vi "winForms keyDownResponse.vi"(4 "searchString":refnum<vi>, 6 "editorType":T1=enum."SigProc", 7 "Ctrl":bool, 8 "error in (no error)":errorcluster, 9 "Char":i16, 10 "VKey":T2, 11 "scintillaRefNum":refnum<k24>) -> (0 "error out":errorcluster, 1 "Discard?":bool)   [LabVIEW 2018]
uses:
  <vilib>/event_ctls.llb/eventvkey.ctl
  C:/ATI_MS_InstrumentControl/dll/ScintillaNET.dll
  dll/ScintillaNET.dll
  winForms editorType.ctl
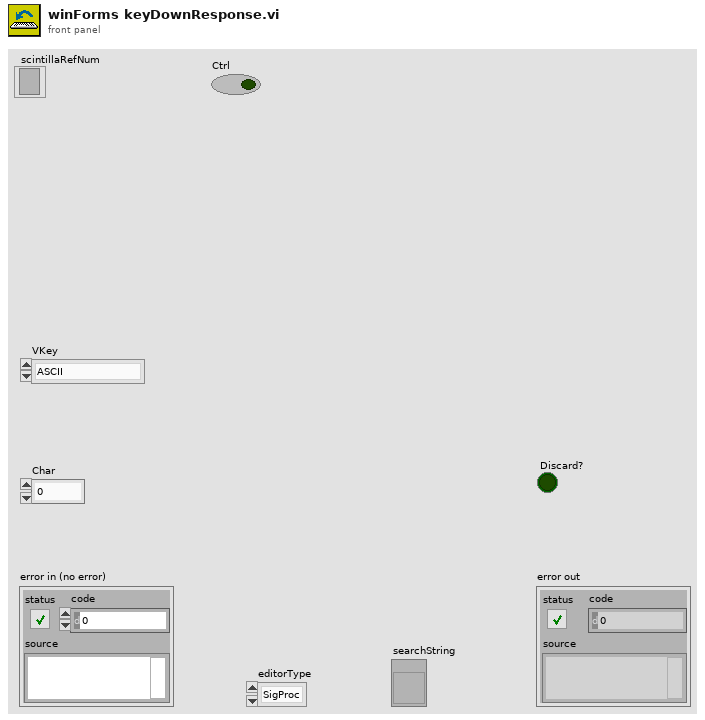
[diagram p1: front panel]
types:
  T1 = typedef "winForms editorType.ctl" = enum16{"Recipe", "SigProc", "Editor"}
  T2 = typedef "eventvkey.ctl" = enum16{"ASCII", "Enter", "Return", "Shift", "Ctrl", "Alt", "Cmd", "Opt", "Caps", "NumLock", "Clear", "Break", "Up", "Down", "Left", "Right", "Insert", "Delete", "Home", "End", "PageUp", "PageDown", "Escape", "Help", "Pause", "ScrollLock", "F1", "F2", "F3", "F4", "F5", "F6", "F7", "F8", "F9", "F10", "F11", "F12", "F13", "F14", "F15", "F16", "F17", "F18", "F19", "F20", "F21", "F22", "F23", "F24", "Play", "VolumeUp", "VolumeDown", "Mute", "Two Byte Char"}
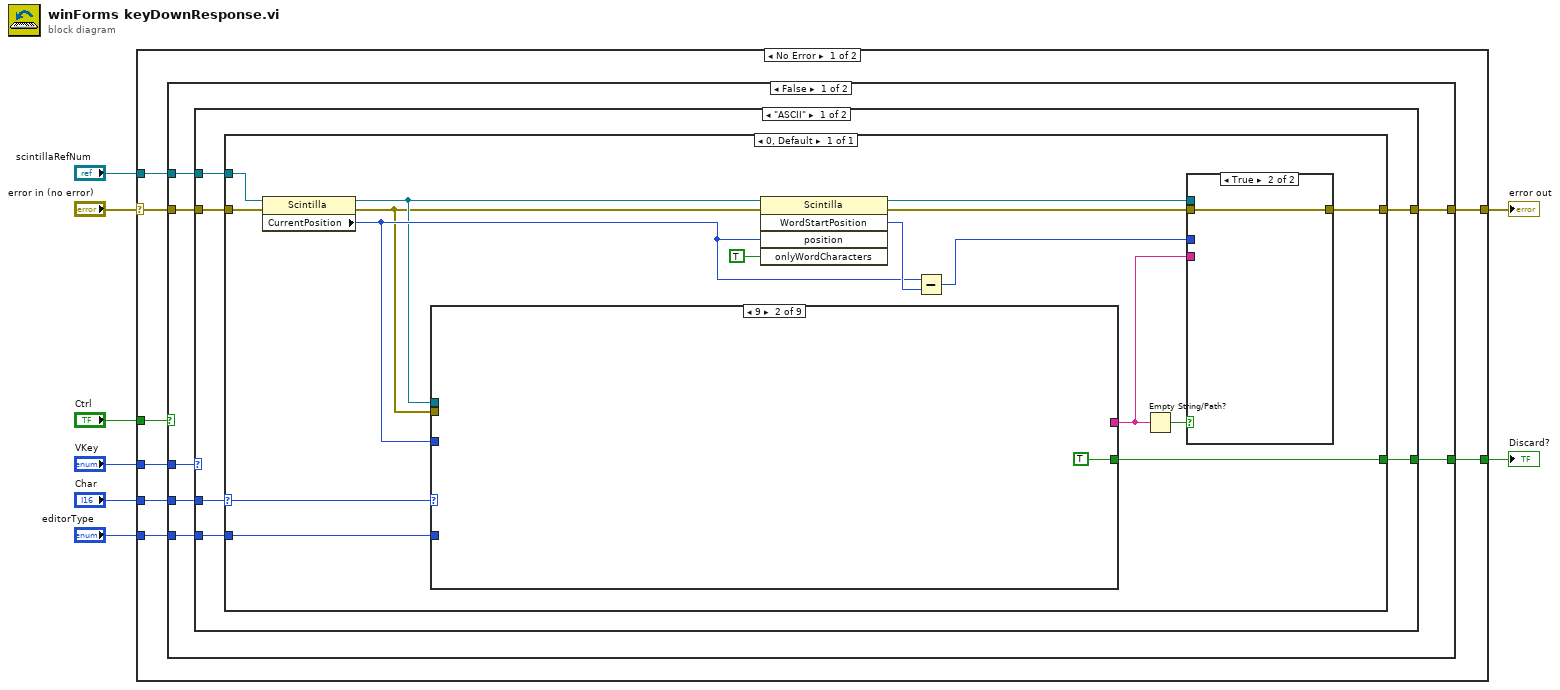
[diagram p0: block diagram]
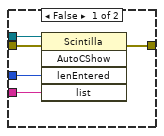
[diagram p2: hidden frame]
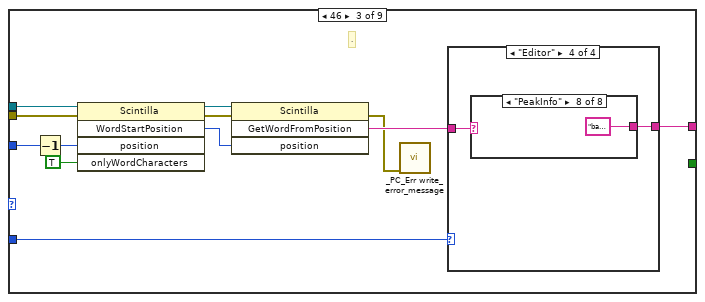
[diagram p4: hidden frame]
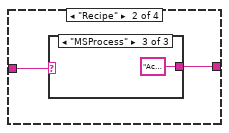
[diagram p6: hidden frame]
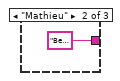
[diagram p8: hidden frame]
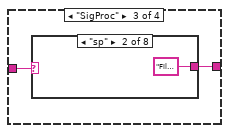
[diagram p9: hidden frame]
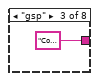
[diagram p11: hidden frame]
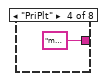
[diagram p12: hidden frame]
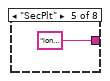
[diagram p13: hidden frame]
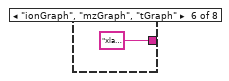
[diagram p14: hidden frame]
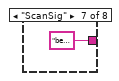
[diagram p15: hidden frame]
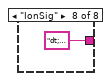
[diagram p16: hidden frame]
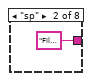
[diagram p18: hidden frame]
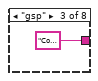
[diagram p19: hidden frame]
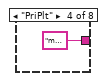
[diagram p20: hidden frame]
diagram:
  n1 = case shown="No Error" "error in (no error)" {
    selector: "error in (no error)" -> [w13 w123]
    tunnel: "VKey" -> [w16 _]
    tunnel: "Char" -> [w15 _]
    tunnel: "scintillaRefNum" -> [w14 _]
    tunnel: [w12 w123] -> w4
    tunnel: [w11 _] -> w3
    tunnel: "editorType" -> [w10 _]
    tunnel: "Ctrl" -> [w9 _]
    frame No Error {
      n2 = case shown="False" w9 {
        tunnel: w16 -> [w23 _]
        tunnel: w15 -> [w22 w110]
        tunnel: w14 -> [w21 w109]
        tunnel: w13 -> [w20 w108]
        tunnel: [w19 w111] -> w12
        tunnel: [w18 TRUE] -> w11
        tunnel: w10 -> [w17 _]
        frame False {
          n3 = case shown="\"ASCII\"" w23 {
            tunnel: w21 -> [w29 _]
            tunnel: w20 -> [w28 w107]
            tunnel: w22 -> [w27 _]
            tunnel: [w26 TRUE] -> w18
            tunnel: [w25 w107] -> w19
            tunnel: w17 -> [w24 _]
            frame "ASCII" {
              n4 = case shown="0, Default" w27 {
                selector: w27 -> [w41]
                tunnel: w29 -> [w37]
                tunnel: w28 -> [w35]
                tunnel: [w30] -> w26
                tunnel: [w36] -> w25
                tunnel: w24 -> [w31]
                frame 0, Default {
                  n5 = property class="Scintilla"(reference=w37, error in=w35) -> (reference out=w33:refnum<k24>, error out=w32:errorcluster, "CurrentPosition"=w34:i32)
                  n6 = case shown="9" w41 {
                    tunnel: [_ _ w64 w87 w90 w93 w96 w100 w103] -> w38
                    tunnel: w34 -> [_ _ w61 _ _ _ _ _ _]
                    tunnel: w33 -> [_ _ w60 _ _ _ _ _ _]
                    tunnel: w32 -> [_ _ w59 _ _ _ _ _ _]
                    tunnel: w31 -> [_ _ w53 w88 w91 w94 w97 w101 w104]
                    tunnel: [_ TRUE _ _ _ _ _ _ _] -> w30
                    frame 0, Default {
                    }
                    frame 9 {
                    }
                    frame 46 {
                      # "."
                      n7 = Decrement(x=w61) -> (x-1=w62:i32)
                      n8 = invoke class="Scintilla" method="WordStartPosition"(reference=w60, error in=w59, "position"=w62, "onlyWordCharacters"=TRUE) -> (reference out=w58:refnum<k24>, error out=w57:errorcluster, "WordStartPosition"=w56:i32)  [unwired: 1 in, 2 out]
                      n9 = invoke class="Scintilla" method="GetWordFromPosition"(reference=w58, error in=w57, "position"=w56) -> (error out=w54:errorcluster, "GetWordFromPosition"=w55:string)  [unwired: 1 in, 2 out]
                      n10 = call "_PC_Err write_error_message.vi"("error in"=w54) -> ()  [unwired: 10 in, 1 out]
                      n11 = case shown="\"Editor\"" w53 {
                        tunnel: [_ w66 w69 w78] -> w64
                        tunnel: w55 -> [_ w65 w70 w79]
                        frame Default {
                        }
                        frame "Recipe" {
                          n12 = case shown="\"MSProcess\"" w65 {
                            tunnel: [_ "Betaofq(q);GetAmp( mz, freq, beta );GetBeta( mz, amp, freq );GetFreq( mz, amp, beta );GetMZ( amp, freq, beta );qofBeta( beta )" "AcqSig( time );AuxScan( auxWfmType, auxStart, iauxCyc, auxCyc, beta, betaScale, auxAmp, auxPulse1, auxPulse2, auxPulseAmp, time );CLFreqScan( targetfreq, time );FGen( amp, freq );Header( ionTrapR0, ionTrapZ0, priRFMaxAmp );IonGate( trialTime, TPH, enableAGC );LaserTrig( trigFreq, phaseDeg, shots );LinearAmpScan( auxWfmType, iauxCyc, beta, betaScale, auxAmp, auxPulse1, auxPulse2, auxPulseAmp, time, amp, continuous );PhaseScan( auxWfmType, auxStart, iauxCyc, auxCyc, beta, betaScale, auxAmp, auxPulse1, auxPulse2, auxPulseAmp, time, freq, stepWidth );PhaseScanII( auxWfmType, auxStart, iauxCyc, auxCyc, beta, betaScale, auxAmp, auxPulse1, auxPulse2, auxPulseAmp, dm, freq, stepWidth );ResetRFPhase( iniPhase );RFStart( freq, amp, wfmType );RFStop();SetDAQ( channel, sampRate );UpdAO( func, val );UpdAuxArbPulses( cycleIni, cycleEnd, pulseInt );UpdConj( iniPhase, conjLen, phaseDiff, fixedLen );UpdDO( func, val );UpdIGVolts( onVolt, offVolt );UpdRFChBias( ch1, ch2, ch3 );UpdRFChFunc( ch1, ch2, ch3 );UpdRFChScale( ch1, ch2, ch3 );Wait( timeout, DI, edge )"] -> w66
                            frame Default {
                            }
                            frame "Mathieu" {
                            }
                            frame "MSProcess" {
                            }
                          }
                        }
                        frame "SigProc" {
                          n13 = case shown="\"sp\"" w70 {
                            tunnel: [_ "Filtering( dt, ydata, ktype, kwidth );MakeKernel( dt, ktype, kwidth );NumRectifier( dt, ydata );NumRectifier_SG( dt, ydata, winwidth );PltAbs( pltData );PltFFT( pltData );PltFiltering( pltData, ktype, kwidth );PltNeg( pltData );PltNumRectifier( pltData );PltNumRectifier_SG( pltData, winwidth )" "Conv1D( kernel, ydata );PltConv1D( kernel , pltData )" "mzGraph;ScanSig;tGraph" "ionGraph;IonSig" "xlabel;ylabel" "beta;dt;xdata;ydata" "dt;ydata"] -> w69
                            frame Default {
                            }
                            frame "sp" {
                            }
                            frame "gsp" {
                            }
                            frame "PriPlt" {
                            }
                            frame "SecPlt" {
                            }
                            frame "ionGraph", "mzGraph", "tGraph" {
                            }
                            frame "ScanSig" {
                            }
                            frame "IonSig" {
                            }
                          }
                        }
                        frame "Editor" {
                          n14 = case shown="\"PeakInfo\"" w79 {
                            tunnel: [_ "Filtering( dt, ydata, ktype, kwidth );MakeKernel( dt, ktype, kwidth );NumRectifier( dt, ydata );NumRectifier_SG( dt, ydata, winwidth );PltAbs( pltData );PltFFT( pltData );PltFiltering( pltData, ktype, kwidth );PltNeg( pltData );PltNumRectifier( pltData );PltNumRectifier_SG( pltData, winwidth )" "Conv1D( kernel, ydata );PltConv1D( kernel , pltData )" "mzGraph;ScanSig;tGraph" "PeakInfo" "xlabel;ylabel" "beta;dt;xdata;ydata" "baseline;halfHeight;xCdata;xLdata;xRdata"] -> w78
                            frame Default {
                            }
                            frame "sp" {
                            }
                            frame "gsp" {
                            }
                            frame "PriPlt" {
                            }
                            frame "PeakPlt" {
                            }
                            frame "ionGraph", "mzGraph", "tGraph" {
                            }
                            frame "ScanSig" {
                            }
                            frame "PeakInfo" {
                            }
                          }
                        }
                      }
                    }
                    frame 71, 103 {
                      # "g,G"
                      n15 = case shown="\"SigProc\"" w88 {
                        tunnel: ["gsp" ("list") _] -> w87
                        frame "SigProc" {
                        }
                        frame Default {
                        }
                      }
                    }
                    frame 73, 105 {
                      # "I,i"
                      n16 = case shown="\"Recipe\"" w91 {
                        tunnel: ["instr" ("list") _] -> w90
                        frame "Recipe" {
                        }
                        frame Default {
                        }
                      }
                    }
                    frame 77, 109 {
                      # "m,M"
                      n17 = case shown="\"Recipe\"" w94 {
                        tunnel: ["Mathieu;MSProcess" ("list") _] -> w93
                        frame "Recipe" {
                        }
                        frame Default {
                        }
                      }
                    }
                    frame 80, 112 {
                      # "p,P"
                      n18 = case shown="\"SigProc\"" w97 {
                        tunnel: ["PriPlt" ("list") "PeakPlt;PriPlt" ("list") _] -> w96
                        frame "SigProc" {
                        }
                        frame "Editor" {
                        }
                        frame Default {
                        }
                      }
                    }
                    frame 83, 115 {
                      # "s,S"
                      n19 = case shown="\"SigProc\"" w101 {
                        tunnel: ["SecPlt;sp" ("list") _] -> w100
                        frame "SigProc" {
                        }
                        frame Default {
                        }
                      }
                    }
                    frame 85, 117 {
                      # "U,u"
                      n20 = case shown="\"Recipe\"" w104 {
                        tunnel: ["user" ("list") _] -> w103
                        frame "Recipe" {
                        }
                        frame Default {
                        }
                      }
                    }
                  }
                  n21 = invoke class="Scintilla" method="WordStartPosition"(reference=w33, error in=w32, "position"=w34, "onlyWordCharacters"=TRUE) -> (reference out=w45:refnum<k24>, error out=w44:errorcluster, "WordStartPosition"=w40:i32)  [unwired: 1 in, 2 out]
                  n22 = Subtract(x=w34, y=w40) -> (x-y=w42:i32)
                  n23 = Empty String/Path?(string/path=w38) -> (empty?=w39:bool)
                  n24 = case shown="True" w39 {
                    tunnel: w45 -> [w50 _]
                    tunnel: w44 -> [w49 w51]
                    tunnel: w42 -> [w48 _]
                    tunnel: w38 -> [w47 _]
                    tunnel: [w46 w51] -> w36
                    frame False {
                      n25 = invoke class="Scintilla" method="AutoCShow"(reference=w50, error in=w49, "lenEntered"=w48, "list"=w47) -> (error out=w46:errorcluster)  [unwired: 1 in, 4 out]
                    }
                    frame True {
                    }
                  }
                }
              }
            }
            frame "Enter", Default {
            }
          }
        }
        frame True {
          n26 = case shown="102" w110 {
            tunnel: w109 -> [w114 w120]
            tunnel: w108 -> [w113 w119]
            tunnel: [w115 w122] -> w111
            frame 0, Default {
              n27 = invoke class="Scintilla" method="BeginUndoAction"(reference=w114, error in=w113) -> (reference out=w116:refnum<k24>, error out=w117:errorcluster)  [unwired: 1 in, 1 out]
              n28 = invoke class="Scintilla" method="EndUndoAction"(reference=w116, error in=w117) -> (error out=w115:errorcluster)  [unwired: 1 in, 2 out]
            }
            frame 102 {
              n29 = invoke class="Scintilla" method="Undo"(reference=w120, error in=w119) -> (error out=w118:errorcluster)  [unwired: 1 in, 2 out]
              n30 = call "winFormsSubVI searchLayout.vi"("error in (no error)"=w118, "searchString"="searchString") -> ("error out"=w122:errorcluster)  [unwired: 9 in]
            }
          }
        }
      }
    }
    frame Error {
    }
  }
  "error out" <- w4
  "Discard?" <- w3
